vi "Image_To_Maze_Array.vi"() -> ()   [LabVIEW 2016]
uses:
  <vilib>/picture/picture.llb/imagedata.ctl
  Controls/Split_Color.ctl
panel:
  in  "Walls to Tunnel":i32=1
  out "Wall Index":i32[](array[numeric])
  out "Array 2":T1[](array[typedef]) {"R" format="%.0x"; "G" format="%.0x"; "B" format="%.0x"}
  out "Is Whites 2":bool[](array[boolean])
  out "Wall Thickness (px) 2":i32
  out "Wall Thickness (px)":i32
  out "Is Whites":bool[](array[boolean])
  out "Array":T1[](array[typedef]) {"R" format="%.0x"; "G" format="%.0x"; "B" format="%.0x"}
  out "Output Array 2":u32[](array[numeric]) format="%06x"
  out "size(s)":i32[](array[numeric])
  out "24-bit pixmap":u32[][](array[numeric]) format="%x"
  out "image data":T2
  in  "Path":path
  # "Height"
  # "Width"
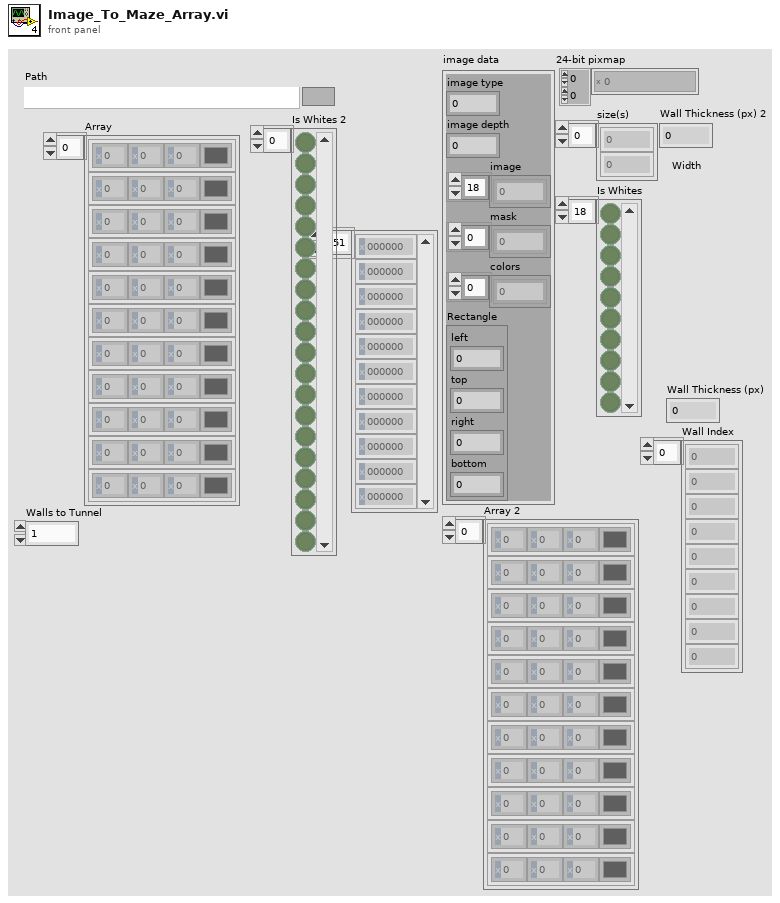
[diagram p1: front panel]
types:
  T1 = typedef "Split_Color.ctl" = cluster{"R":u8, "G":u8, "B":u8, "Color Box":u32}
  T2 = typedef "imagedata.ctl" = cluster{"image type":i32, "image depth":i32, "image":u8[], "mask":u8[], "colors":u32[], "Rectangle":cluster{"left":i16, "top":i16, "right":i16, "bottom":i16}}
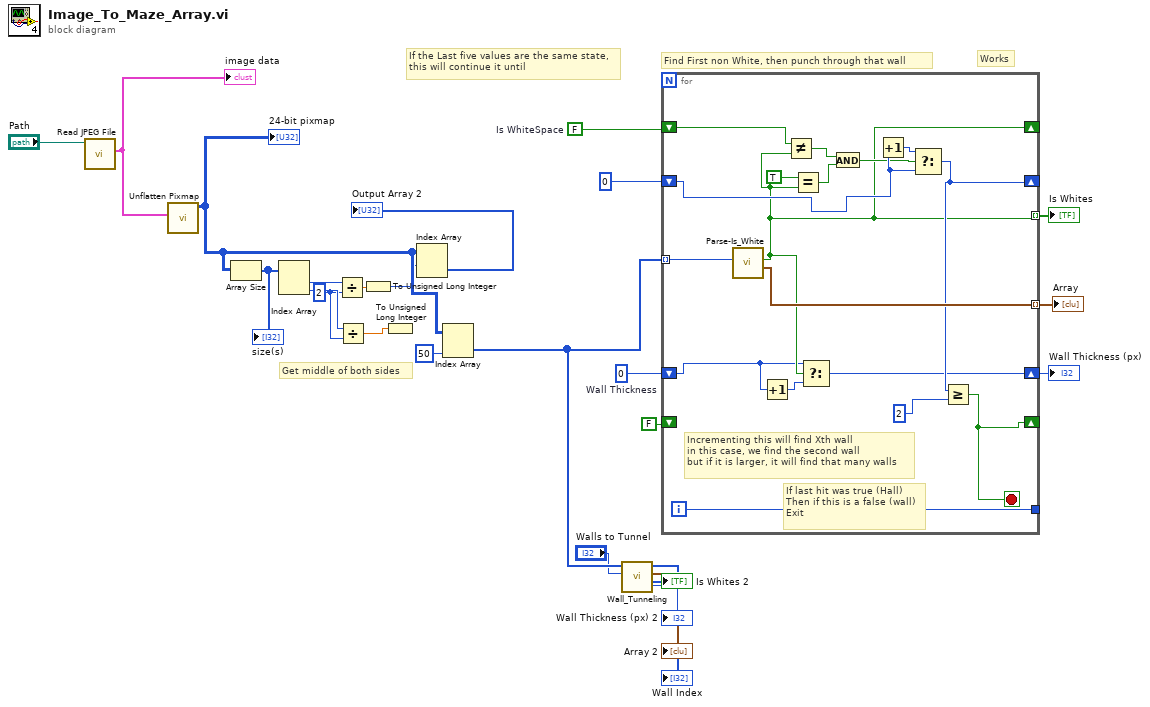
[diagram p0: block diagram]
diagram:
  w8 = 0  # Wall Thickness
  w11 = FALSE  # Is WhiteSpace
  w20 = 2 ("y")
  # "Works"
  # "Find First non White, then punch through that wall"
  # "If the Last five values are the same state,\nthis will continue it until"
  # "Get middle of both sides"
  n1 = call <vilib>:"Read JPEG File.vi"("path to JPEG file"="Path") -> ("image data"=w24:T2)  [unwired: 8 in, 2 out]
  "image data" <- w24
  n2 = call <vilib>:"Unflatten Pixmap.vi"("image data"=w24) -> ("24-bit pixmap"=w17:u32[][])  [unwired: 4 in, 6 out]
  "24-bit pixmap" <- w17
  n3 = Array Size(array=w17) -> (size(s)=w23:i32[])
  "size(s)" <- w23
  n4 = Index Array(array=w23) -> (element #1=w22:i32, element #2=w21:i32)  [unwired: 2 in]
  n5 = Divide(x=w22, y=w20) -> (x/y=w19:dbl)
  n6 = Divide(x=w21, y=w20) -> (x/y=w18:dbl)
  n7 = To Unsigned Long Integer(number=w19) -> (unsigned 32bit integer=w16:u32)
  n8 = To Unsigned Long Integer(number=w18) -> ()  [unwired: 1 out]
  n9 = Index Array(array=w17, index (row)=w16) -> (element=→"Output Array 2":u32[])  [unwired: 1 in]
  n10 = Index Array(array=w17, index (col)=50 ("disabled index (col)")) -> (element=w6:u32[])  [unwired: 1 in]
  n11 = call "Wall_Tunneling.vi"("Walls to Tunnel"="Walls to Tunnel", "Line to Parse"=w6) -> ("Tile Type"=→"Is Whites 2":u16[], "Array"=→"Array 2":T1[], "Wall Index"=→"Wall Index":i32[], "Wall Thickness (px)"=→"Wall Thickness (px) 2":i32)  [unwired: 6 in]
  n12 = for {
    tunnel: w6 -> [w42] mode=indexing
    shift-right: [w30] -> _
    shift-left: w11 -> [w39]
    shift-right: [w32] -> _
    shift-left: FALSE -> [_]
    tunnel: [w41] -> w12 mode=indexing
    shift-right: [w33] -> _
    shift-left: 0 -> [w35]
    tunnel: [w30] -> w9 mode=indexing
    shift-right: [w27] -> w7
    shift-left: w8 -> [w29]
    tunnel: [w26] -> _
    i -> [w26]
    stop <- w32 stop-if-true
    # "Incrementing this will find Xth wall\nin this case, we find the second wall\nbut if it is larger, it will find that many walls"
    # "If last hit was true (Hall)\nThen if this is a false (wall)\nExit"
    n13 = call "Parse-Is_White.vi"("Color"=w42) -> ("Color Cluster"=w41:T1, "Is White"=w30:bool)  [unwired: 8 in, 1 out]
    n14 = Increment(x=w29) -> (x+1=w28:i32)
    n15 = Not Equal?(x=w39, y=w30) -> (x != y?=w38:bool)
    n16 = Equal?(x=TRUE, y=w30) -> (x = y?=w37:bool)
    n17 = Select(t=w29, s=w30, f=w28) -> (s? t:f=w27:i32)
    n18 = And(x=w38, y=w37) -> (x .and. y?=w31:bool)
    n19 = Increment(x=w35) -> (x+1=w36:i32)
    n20 = Select(t=w36, s=w31, f=w35) -> (s? t:f=w33:i32)
    n21 = Greater Or Equal?(x=w33, y=2) -> (x >= y?=w32:bool)
  }
  "Array" <- w12
  "Is Whites" <- w9
  "Wall Thickness (px)" <- w7
